vi "TCPtaskhandle.vi"(6 "心跳包":refnum<vi>, 9 "配置信息":refnum<vi>, 10 "状态信息":refnum<vi>, 11 "通信状态":refnum<vi>) -> ()   [LabVIEW 2016, in "数据传输系统-06.lvlib"]
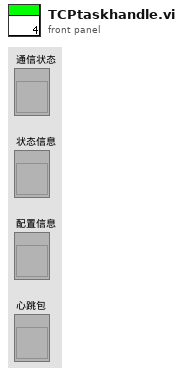
[diagram p1: front panel]
types:
  T1 = cluster{"枚举":enum16{"打开连接", "发送数据", "读取数据", "数据处理", "关闭连接"}, "发送报文":string}
  T2 = cluster{"setini":string, "sysini":string, "hechaini":string, "actualwrite":string, "actualread":string, "datasent":string, "反控命令信息队列":string, "反控与仪器交互":string}
  T3 = cluster{"站点":string, "设备":string, "IP":string, "PORT":string, "MN":string, "PW":string}
  T4 = cluster{"1st Error to Convert ":i32, "步骤 ":enum16{"打开连接", "发送数据", "读取数据", "数据处理", "关闭连接"}, "元素":string, "TCP服务端掉线计数":i32, "TCP掉线时间节点":string}
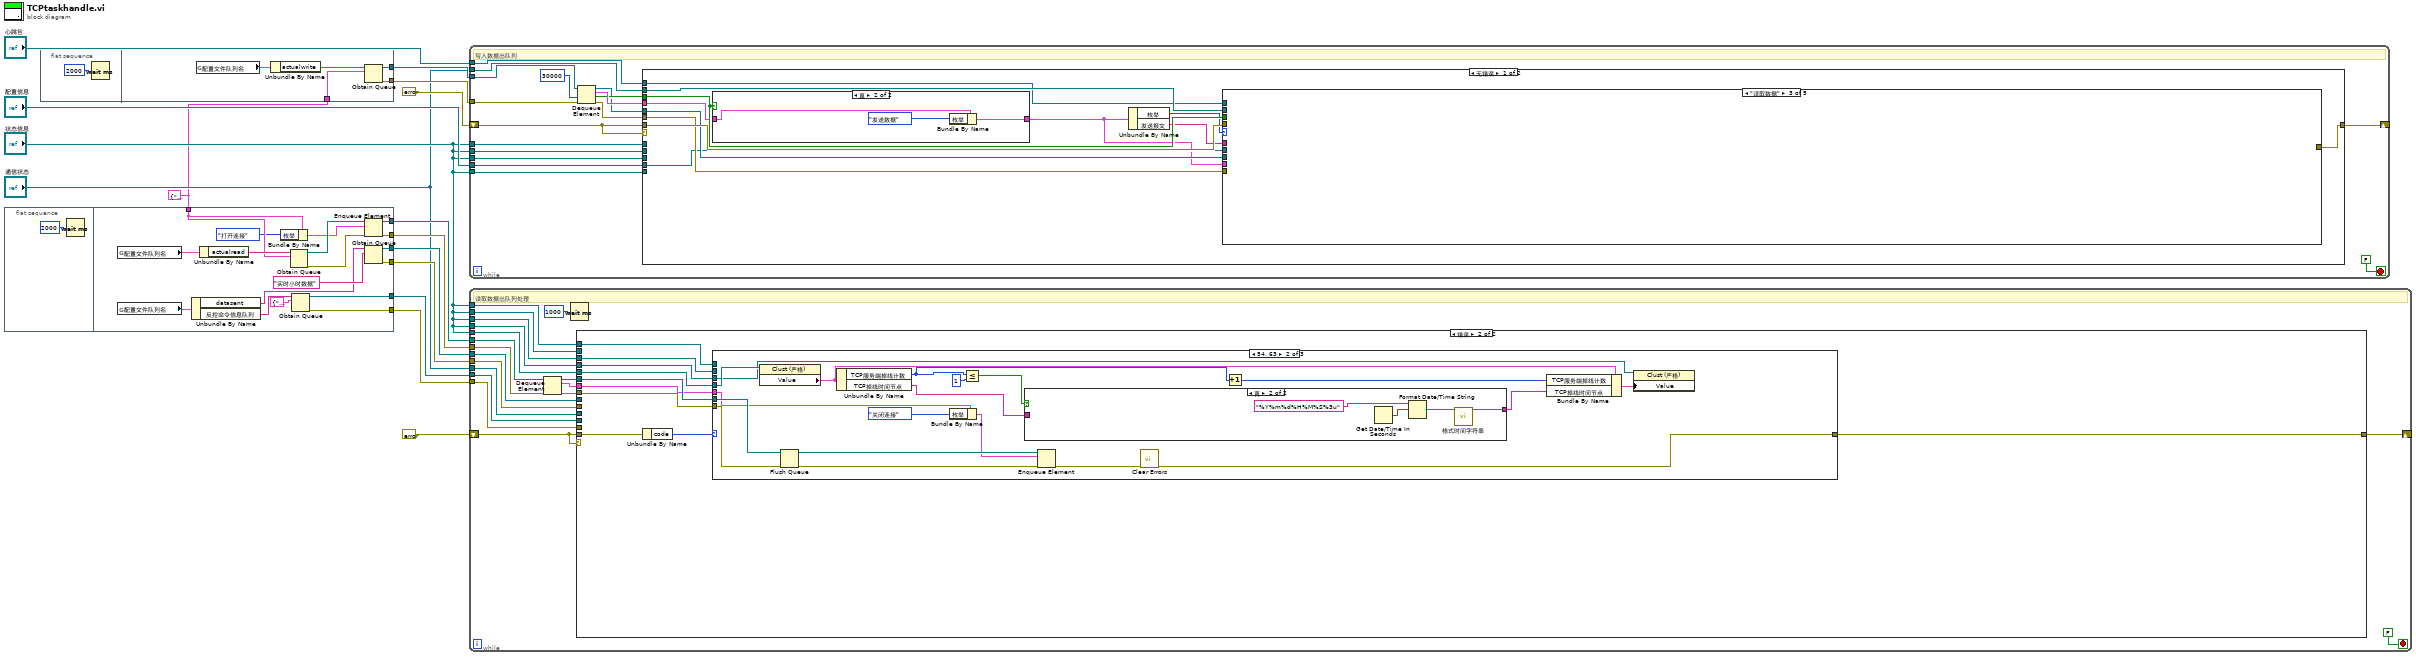
[diagram p0: block diagram]
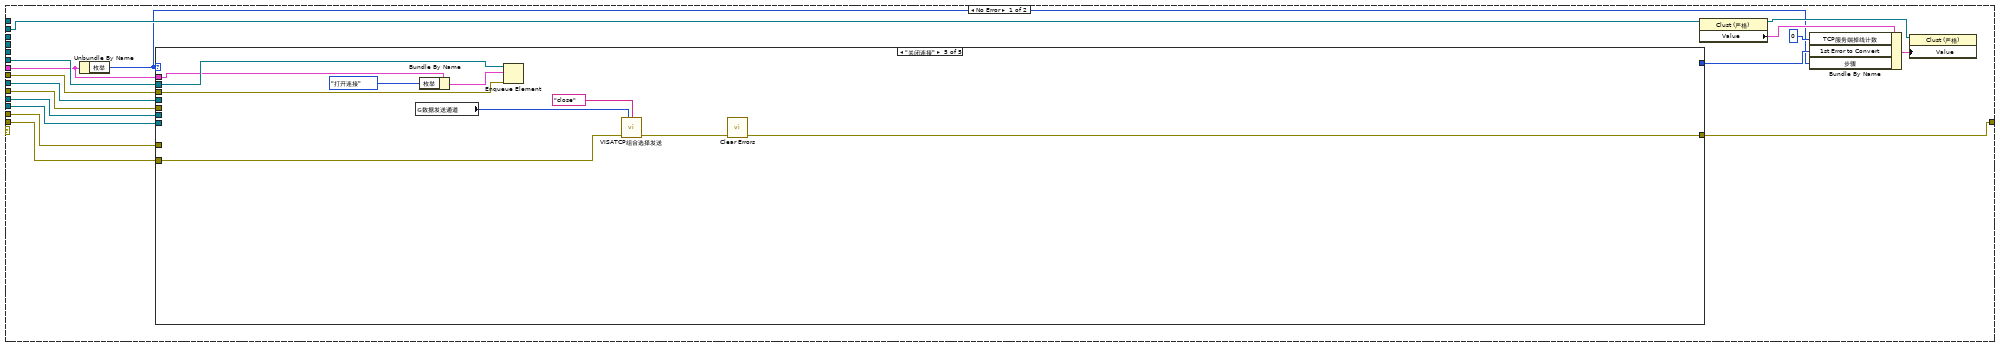
[diagram p2: hidden frame]
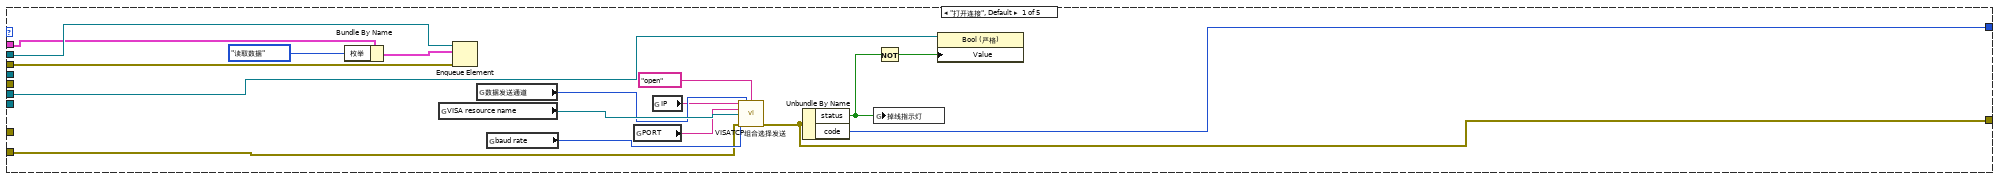
[diagram p3: hidden frame]
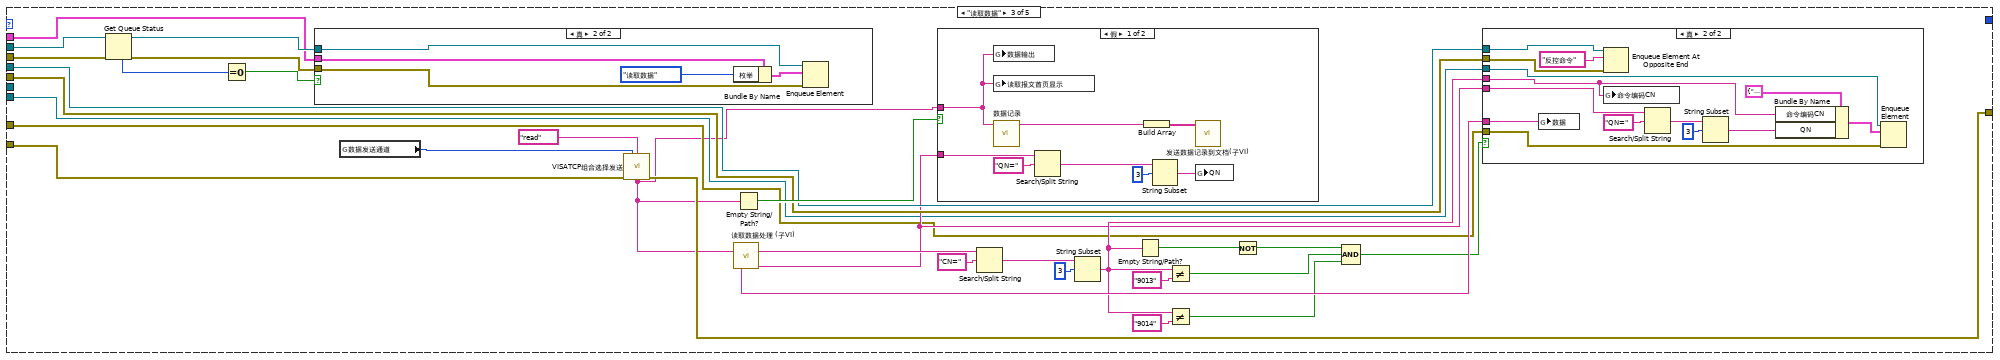
[diagram p5: hidden frame]
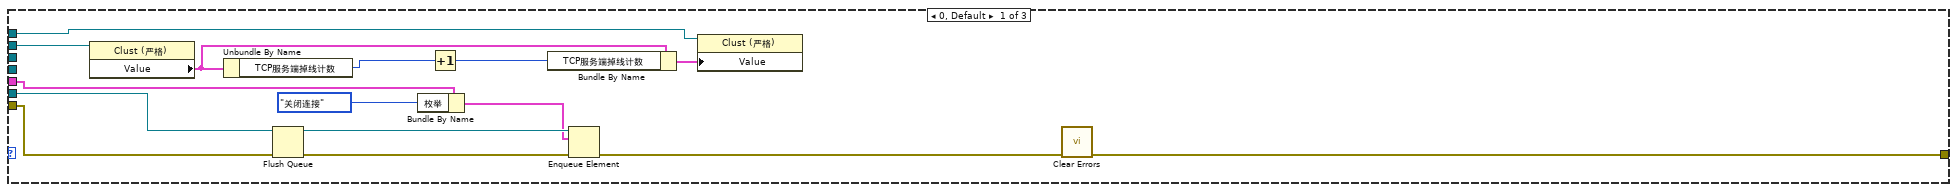
[diagram p10: hidden frame]
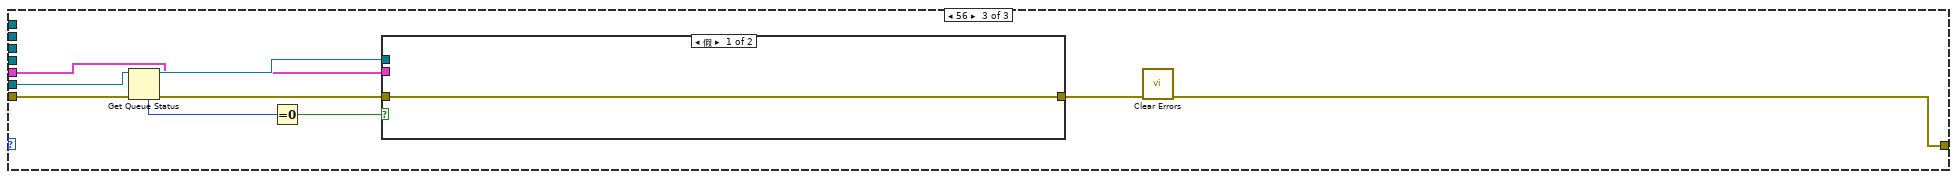
[diagram p12: hidden frame]
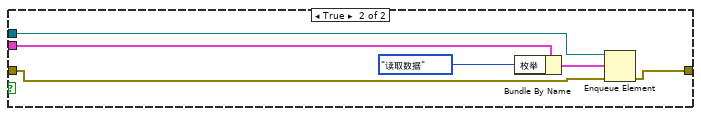
[diagram p13: hidden frame]
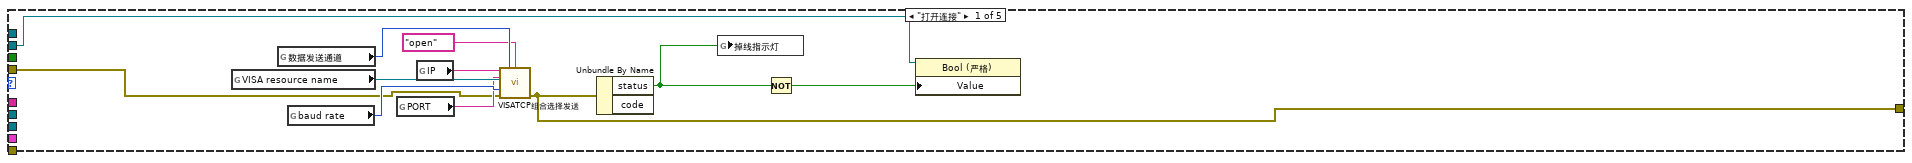
[diagram p14: hidden frame]
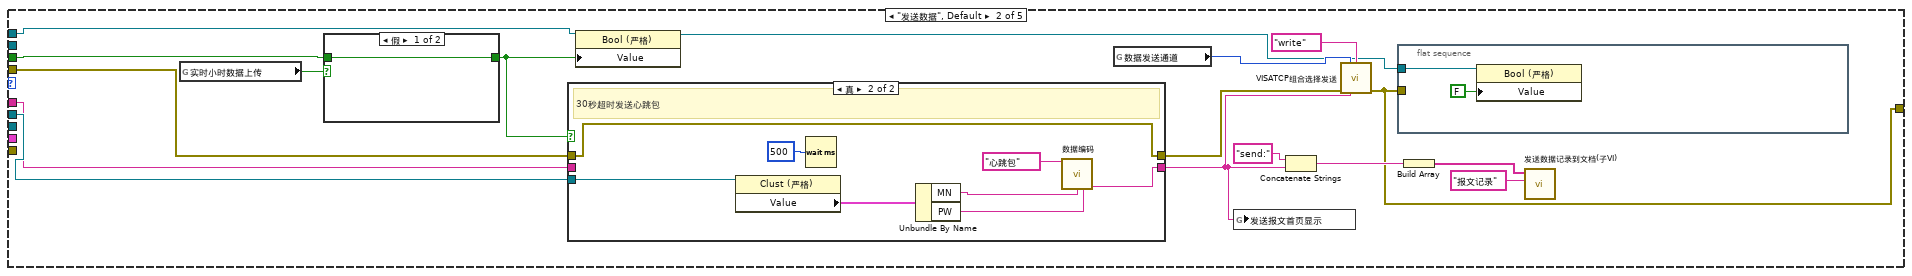
[diagram p15: hidden frame]
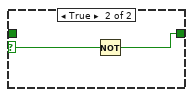
[diagram p17: hidden frame]
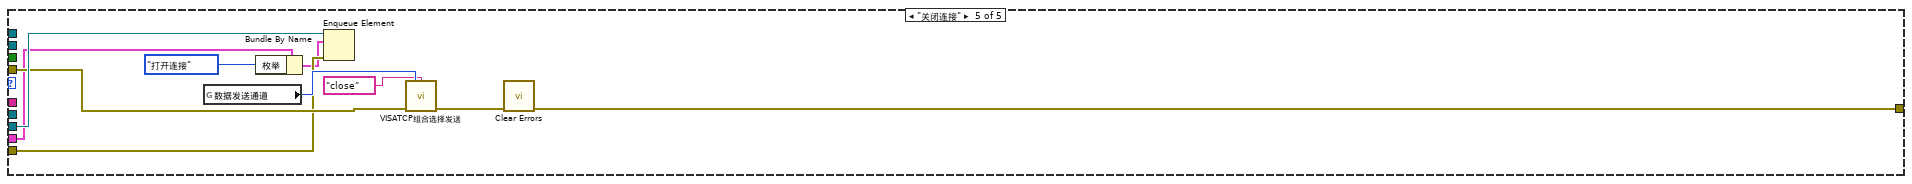
[diagram p19: hidden frame]
diagram:
  w1 = T1 {"枚举"=enum."打开连接", "发送报文"=""} ("data")
  n1 = flat-sequence {
    tunnel: [w33] -> w9
    tunnel: [w32] -> w10
    tunnel: [w30] -> w12
    tunnel: [w29] -> w13
    tunnel: [w27] -> w14
    tunnel: [w26] -> w15
    tunnel: w1 -> [w19]
    frame #0 {
      n2 = Wait (ms)(milliseconds to wait=u32 2000 ("等待时间（毫秒）")) -> ()  [unwired: 1 out]
    }
    frame #1 {
      n3 = global read "断电保存全局.vi" "配置文件队列名"() -> (w24:T2)
      n4 = global read "断电保存全局.vi" "配置文件队列名"() -> (w22:T2)
      n5 = Unbundle By Name(w22) -> ("datasent"=w21:string, "反控命令信息队列"=w20:string)
      n6 = Unbundle By Name(w24) -> ("actualread"=w23:string)
      n7 = Bundle By Name(cluster=w19, "枚举"=enum16{"打开连接", "发送数据", "读取数据", "数据处理", "关闭连接"}."打开连接") -> (w17:T1)
      n8 = Obtain Queue(name (unnamed)=w23, element data type=w19) -> (queue out=w34:refnum<queue>, error out=w31:errorcluster)  [unwired: 3 in, 1 out]
      n9 = Obtain Queue(name (unnamed)=w20, element data type=cluster{"命令编码CN":string, "QN":string} {"命令编码CN"="", "QN"=""}) -> (queue out=w27:refnum<queue>, error out=w26:errorcluster)  [unwired: 3 in, 1 out]
      n10 = Enqueue Element(queue=w34, element=w17, error in (no error)=w31) -> (queue out=w33:refnum<queue>, error out=w32:errorcluster)  [unwired: 1 in, 1 out]
      n11 = Obtain Queue(name (unnamed)=w21, element data type="实时小时数据" ("元素")) -> (queue out=w30:refnum<queue>, error out=w29:errorcluster)  [unwired: 3 in, 1 out]
    }
  }
  n12 = flat-sequence {
    tunnel: [w40] -> w6
    tunnel: [w39] -> w7
    tunnel: w1 -> [w36]
    frame #0 {
      n13 = Wait (ms)(milliseconds to wait=u32 2000 ("等待时间（毫秒）")) -> ()  [unwired: 1 out]
    }
    frame #1 {
      n14 = global read "断电保存全局.vi" "配置文件队列名"() -> (w38:T2)
      n15 = Unbundle By Name(w38) -> ("actualwrite"=w37:string)
      n16 = Obtain Queue(name (unnamed)=w37, element data type=w36) -> (queue out=w40:refnum<queue>, error out=w39:errorcluster)  [unwired: 3 in, 1 out]
    }
  }
  n17 = while {
    tunnel: w6 -> [w56]
    tunnel: w7 -> [w55]
    shift-right: [w51] -> _
    shift-left: errorcluster {"status"=FALSE, "code"=0, "source"=""} ("error out") -> [w50]
    tunnel: "通信状态" -> [w47]
    tunnel: "配置信息" -> [w46]
    tunnel: "心跳包" -> [w45]
    tunnel: "状态信息" -> [w44]
    tunnel: "状态信息" -> [w43]
    tunnel: "状态信息" -> [w42]
    tunnel: "状态信息" -> [w41]
    stop <- FALSE stop-if-true
    # "写入数据出队列"
    n18 = Dequeue Element(queue=w56, timeout in ms (-1)=30000 ("超时毫秒(-1)"), error in (no error)=w55) -> (queue out=w49:refnum<queue>, element=w53:T1, timed out?=w52:bool, error out=w48:errorcluster)
    n19 = case shown="无错误" w50 {
      tunnel: w53 -> [w64 w127]
      tunnel: w52 -> [w65 _]
      tunnel: [w69 w132] -> w51
      tunnel: w50 -> [w68 w136]
      tunnel: w49 -> [w67 w134]
      tunnel: w48 -> [w66 w133]
      tunnel: w47 -> [w63 _]
      tunnel: w46 -> [w62 _]
      tunnel: w45 -> [w61 _]
      tunnel: w44 -> [_ w131]
      tunnel: w43 -> [_ w130]
      tunnel: w42 -> [_ w129]
      tunnel: w41 -> [_ w128]
      frame No Error {
        n20 = case shown="真" w65 {
          tunnel: [w123 w124] -> w58
          tunnel: w64 -> [w123 w126]
          frame False {
          }
          frame True {
            n21 = Bundle By Name(cluster=w126, "枚举"=enum16{"打开连接", "发送数据", "读取数据", "数据处理", "关闭连接"}."发送数据") -> (w124:T1)
          }
        }
        n22 = Unbundle By Name(w58) -> ("枚举"=w60:enum16{"打开连接", "发送数据", "读取数据", "数据处理", "关闭连接"}, "发送报文"=w59:string)
        n23 = case shown="\"读取数据\"" w60 {
          tunnel: w65 -> [_ w87 _ _ _]
          tunnel: [w72 w90 _ _ w117] -> w69
          tunnel: w68 -> [w74 w95 _ _ w118]
          tunnel: w67 -> [_ _ _ _ w119]
          tunnel: w66 -> [_ _ _ _ w116]
          tunnel: w63 -> [w70 _ _ _ _]
          tunnel: w62 -> [_ w86 _ _ _]
          tunnel: w61 -> [_ w84 _ _ _]
          tunnel: w59 -> [_ w82 _ _ _]
          tunnel: w58 -> [_ _ _ _ w114]
          frame "打开连接" {
            n24 = global read "断电保存全局.vi" "VISA resource name"() -> (w80:refnum<visa-resource-name>)
            n25 = global read "断电保存全局.vi" "数据发送通道"() -> (w77:enum16{"TCP", "VISA"})
            n26 = global read "断电保存全局.vi" "baud rate"() -> (w79:u32)
            n27 = global read "断电保存全局.vi" "PORT"() -> (w78:string)
            n28 = global read "断电保存全局.vi" "IP"() -> (w76:string)
            n29 = call "VISATCP组合选择发送.vi"("IP"=w76, "数据发送通道"=w77, "命令"="open", "PORT"=w78, "VISA resource name"=w80, "baud rate"=w79, "error in (no error)"=w74) -> ("错误输出"=w72:errorcluster)  [unwired: 5 in, 3 out]
            n30 = Unbundle By Name(w72) -> ("status"=w71:bool)  [unwired: 1 out]
            n31 = global write "全局 数据发送重叠.vi" "掉线指示灯"(w71) -> ()
            n32 = Not(x=w71) -> (.not. x?=w73:bool)
            n33 = property class="Bool (严格)"(reference=w70, "Value"=w73) -> ()  [unwired: 1 in, 2 out]
          }
          frame "发送数据", Default {
            n34 = global read "全局1.vi" "实时小时数据上传"() -> (w88:bool)
            n35 = case shown="假" w88 {
              selector: w88 -> [_ w112]
              tunnel: w87 -> [w110 _]
              tunnel: [w110 w111] -> w85
              frame False {
              }
              frame True {
                n36 = Not(x=w112) -> (.not. x?=w111:bool)
              }
            }
            n37 = case shown="真" w85 {
              tunnel: [w100 w104] -> w81
              tunnel: w95 -> [w101 w105]
              tunnel: [w101 w105] -> w94
              tunnel: w86 -> [_ w102]
              tunnel: w82 -> [w100 _]
              frame False {
                # "事件触发发送数据"
              }
              frame True {
                # "30秒超时发送心跳包"
                n38 = property class="Clust (严格)"(reference=w102) -> ("Value"=w108:T3)  [unwired: 1 in, 2 out]
                n39 = Wait (ms)(milliseconds to wait=u32 500 ("等待时间（毫秒）")) -> ()  [unwired: 1 out]
                n40 = Unbundle By Name(w108) -> ("MN"=w107:string, "PW"=w106:string)
                n41 = call "数据编码.vi"("table输入"="心跳包", "MN"=w107, "PW"=w106) -> ("通讯包字符串"=w104:string)  [unwired: 11 in, 1 out]
              }
            }
            n42 = property class="Bool (严格)"(reference=w84, "Value"=w85) -> (reference out=w83:refnum<vi>)  [unwired: 1 in, 1 out]
            n43 = global read "断电保存全局.vi" "数据发送通道"() -> (w96:enum16{"TCP", "VISA"})
            n44 = global write "全局1.vi" "发送报文首页显示"(w81) -> ()
            n45 = Concatenate Strings("send:" ("字符串"), w81) -> (w91:string)
            n46 = call "VISATCP组合选择发送.vi"("数据发送通道"=w96, "命令"="write", "error in (no error)"=w94, "写入缓冲区"=w81) -> ("错误输出"=w90:errorcluster)  [unwired: 8 in, 3 out]
            n47 = flat-sequence {
              tunnel: w90 -> [_]
              tunnel: w83 -> [w98]
              frame #0 {
                n48 = property class="Bool (严格)"(reference=w98, "Value"=FALSE ("心跳包")) -> ()  [unwired: 1 in, 2 out]
              }
            }
            n49 = Build Array(w91) -> (w93:string[])
            n50 = call "发送数据记录到文档(子VI).vi"("字符串"="报文记录", "数组"=w93) -> ()  [unwired: 8 in, 1 out]
          }
          frame "读取数据" {
          }
          frame "数据处理" {
          }
          frame "关闭连接" {
            n51 = global read "断电保存全局.vi" "数据发送通道"() -> (w121:enum16{"TCP", "VISA"})
            n52 = Bundle By Name(cluster=w114, "枚举"=enum16{"打开连接", "发送数据", "读取数据", "数据处理", "关闭连接"}."打开连接") -> (w113:T1)
            n53 = Enqueue Element(queue=w119, element=w113, error in (no error)=w116) -> ()  [unwired: 1 in, 3 out]
            n54 = call "VISATCP组合选择发送.vi"("数据发送通道"=w121, "命令"="close", "error in (no error)"=w118) -> ("错误输出"=w122:errorcluster)  [unwired: 9 in, 3 out]
            n55 = call <vilib>:"Clear Errors.vi"("error in (no error)"=w122) -> ("error out"=w117:errorcluster)  [unwired: 5 in, 1 out]
          }
        }
      }
      frame Error {
        n56 = Unbundle By Name(w136) -> ("code"=w135:i32)
        n57 = case shown="0, 默认" w135 {
          tunnel: w134 -> [w148 w168 w179]
          tunnel: w133 -> [w147 w167 w178]
          tunnel: [w146 w165 w177] -> w132
          tunnel: w131 -> [w141 _ _]
          tunnel: w130 -> [w140 _ _]
          tunnel: w129 -> [_ w156 _]
          tunnel: w128 -> [_ w155 _]
          tunnel: w127 -> [w138 w154 _]
          frame 0, Default {
            n58 = property class="Clust (严格)"(reference=w141) -> ("Value"=w145:T4)  [unwired: 1 in, 2 out]
            n59 = Unbundle By Name(w145) -> ("TCP服务端掉线计数"=w143:i32)
            n60 = Flush Queue(queue=w148, error in (no error)=w147) -> (queue out=w149:refnum<queue>, error out=w150:errorcluster)  [unwired: 1 out]
            n61 = Bundle By Name(cluster=w138, "枚举"=enum16{"打开连接", "发送数据", "读取数据", "数据处理", "关闭连接"}."关闭连接") -> (w137:T1)
            n62 = Increment(x=w143) -> (x+1=w144:i32)
            n63 = Bundle By Name(cluster=w145, "TCP服务端掉线计数"=w144) -> (w142:T4)
            n64 = Enqueue Element(queue=w149, element=w137, error in (no error)=w150) -> (error out=w151:errorcluster)  [unwired: 1 in, 2 out]
            n65 = property class="Clust (严格)"(reference=w140, "Value"=w142) -> ()  [unwired: 1 in, 2 out]
            n66 = call <vilib>:"Clear Errors.vi"("error in (no error)"=w151) -> ("error out"=w146:errorcluster)  [unwired: 5 in, 1 out]
          }
          frame 54, 63 {
            n67 = property class="Clust (严格)"(reference=w156) -> ("Value"=w160:T4)  [unwired: 1 in, 2 out]
            n68 = Flush Queue(queue=w168, error in (no error)=w167) -> (queue out=w169:refnum<queue>, error out=w170:errorcluster)  [unwired: 1 out]
            n69 = Unbundle By Name(w160) -> ("TCP服务端掉线计数"=w164:i32, "TCP掉线时间节点"=w157:string)
            n70 = Bundle By Name(cluster=w154, "枚举"=enum16{"打开连接", "发送数据", "读取数据", "数据处理", "关闭连接"}."关闭连接") -> (w152:T1)
            n71 = Less Or Equal?(x=w164, y=1) -> (x <= y?=w162:bool)
            n72 = case shown="真" w162 {
              tunnel: [w171 w172] -> w161
              tunnel: w157 -> [w171 _]
              frame False {
              }
              frame True {
                n73 = Get Date/Time In Seconds() -> (seconds since 1Jan1904=w173:timestamp)
                n74 = Format Date/Time String(time format string (%c)="%Y%m%d%H%M%S%3u" ("时间格式字符串(%c)"), seconds (now)=w173) -> (date/time string=w175:string)  [unwired: 1 in]
                n75 = call "格式时间字符串.vi"("字符串"=w175) -> ("连接的字符串"=w172:string)  [unwired: 10 in]
              }
            }
            n76 = Enqueue Element(queue=w169, element=w152, error in (no error)=w170) -> (error out=w166:errorcluster)  [unwired: 1 in, 2 out]
            n77 = call <vilib>:"Clear Errors.vi"("error in (no error)"=w166) -> ("error out"=w165:errorcluster)  [unwired: 5 in, 1 out]
            n78 = Increment(x=w164) -> (x+1=w159:i32)
            n79 = Bundle By Name(cluster=w160, "TCP服务端掉线计数"=w159, "TCP掉线时间节点"=w161) -> (w158:T4)
            n80 = property class="Clust (严格)"(reference=w155, "Value"=w158) -> ()  [unwired: 1 in, 2 out]
          }
          frame 56 {
            n81 = Flush Queue(queue=w179, error in (no error)=w178) -> (error out=w176:errorcluster)  [unwired: 2 out]
            n82 = call <vilib>:"Clear Errors.vi"("error in (no error)"=w176) -> ("error out"=w177:errorcluster)  [unwired: 5 in, 1 out]
          }
        }
      }
    }
  }
  n83 = while {
    tunnel: w9 -> [w198]
    tunnel: w10 -> [w197]
    shift-right: [w194] -> _
    shift-left: errorcluster {"status"=FALSE, "code"=0, "source"=""} ("error out") -> [w193]
    tunnel: w12 -> [w189]
    tunnel: w13 -> [w188]
    tunnel: w14 -> [w187]
    tunnel: w15 -> [w186]
    tunnel: "状态信息" -> [w185]
    tunnel: "状态信息" -> [w184]
    tunnel: "状态信息" -> [w183]
    tunnel: "状态信息" -> [w182]
    tunnel: "状态信息" -> [w181]
    tunnel: "通信状态" -> [w180]
    stop <- FALSE stop-if-true
    # "读取数据出队列处理"
    n84 = Dequeue Element(queue=w198, error in (no error)=w197) -> (queue out=w192:refnum<queue>, element=w195:T1, error out=w191:errorcluster)  [unwired: 1 in, 1 out]
    n85 = Wait (ms)(milliseconds to wait=u32 1000 ("等待时间（毫秒）")) -> ()  [unwired: 1 out]
    n86 = case shown="错误" w193 {
      tunnel: w195 -> [w199 w301]
      tunnel: [w215 w306] -> w194
      tunnel: w193 -> [w214 w310]
      tunnel: w192 -> [w213 w308]
      tunnel: w191 -> [w212 w307]
      tunnel: w189 -> [w208 _]
      tunnel: w188 -> [w207 _]
      tunnel: w187 -> [w206 _]
      tunnel: w186 -> [w205 _]
      tunnel: w185 -> [w204 _]
      tunnel: w184 -> [_ w305]
      tunnel: w183 -> [_ w304]
      tunnel: w182 -> [_ w303]
      tunnel: w181 -> [_ w302]
      tunnel: w180 -> [w201 _]
      frame No Error {
        n87 = Unbundle By Name(w199) -> ("枚举"=w200:enum16{"打开连接", "发送数据", "读取数据", "数据处理", "关闭连接"})
        n88 = case shown="\"关闭连接\"" w200 {
          tunnel: [w226 _ w260 _ w296] -> w215
          tunnel: w214 -> [w225 _ w263 _ w297]
          tunnel: w213 -> [w224 _ w255 _ w295]
          tunnel: w212 -> [w223 _ w254 _ w294]
          tunnel: [w222 _ _ _ _] -> w210
          tunnel: w208 -> [_ _ w248 _ _]
          tunnel: w207 -> [_ _ w247 _ _]
          tunnel: w206 -> [_ _ w236 _ _]
          tunnel: w205 -> [_ _ w235 _ _]
          tunnel: w201 -> [w220 _ _ _ _]
          tunnel: w199 -> [w217 _ w233 _ w291]
          frame "打开连接", Default {
            n89 = Bundle By Name(cluster=w217, "枚举"=enum16{"打开连接", "发送数据", "读取数据", "数据处理", "关闭连接"}."读取数据") -> (w216:T1)
            n90 = global read "断电保存全局.vi" "VISA resource name"() -> (w232:refnum<visa-resource-name>)
            n91 = Enqueue Element(queue=w224, element=w216, error in (no error)=w223) -> ()  [unwired: 1 in, 3 out]
            n92 = global read "断电保存全局.vi" "数据发送通道"() -> (w229:enum16{"TCP", "VISA"})
            n93 = global read "断电保存全局.vi" "baud rate"() -> (w231:u32)
            n94 = global read "断电保存全局.vi" "PORT"() -> (w230:string)
            n95 = global read "断电保存全局.vi" "IP"() -> (w228:string)
            n96 = call "VISATCP组合选择发送.vi"("IP"=w228, "数据发送通道"=w229, "命令"="open", "PORT"=w230, "VISA resource name"=w232, "baud rate"=w231, "error in (no error)"=w225) -> ("错误输出"=w226:errorcluster)  [unwired: 5 in, 3 out]
            n97 = Unbundle By Name(w226) -> ("status"=w221:bool, "code"=w222:i32)
            n98 = global write "全局 数据发送重叠.vi" "掉线指示灯"(w221) -> ()
            n99 = Not(x=w221) -> (.not. x?=w219:bool)
            n100 = property class="Bool (严格)"(reference=w220, "Value"=w219) -> ()  [unwired: 1 in, 2 out]
          }
          frame "发送数据" {
          }
          frame "读取数据" {
            n101 = Get Queue Status(queue=w255, error in (no error)=w254) -> (queue out=w251:refnum<queue>, error out=w250:errorcluster, # elements in queue=w253:i32)  [unwired: 1 in, 5 out]
            n102 = Equal To 0?(x=w253) -> (x = 0?=w252:bool)
            n103 = case shown="真" w252 {
              tunnel: w251 -> [_ w290]
              tunnel: w250 -> [_ w289]
              tunnel: w233 -> [_ w288]
              frame False {
              }
              frame True {
                n104 = Bundle By Name(cluster=w288, "枚举"=enum16{"打开连接", "发送数据", "读取数据", "数据处理", "关闭连接"}."读取数据") -> (w286:T1)
                n105 = Enqueue Element(queue=w290, element=w286, error in (no error)=w289) -> ()  [unwired: 1 in, 3 out]
              }
            }
            n106 = global read "断电保存全局.vi" "数据发送通道"() -> (w262:enum16{"TCP", "VISA"})
            n107 = call "VISATCP组合选择发送.vi"("数据发送通道"=w262, "命令"="read", "error in (no error)"=w263) -> ("读取缓冲区"=w234:string, "错误输出"=w260:errorcluster)  [unwired: 9 in, 2 out]
            n108 = call "读取数据处理 (子VI).vi"("data out"=w234) -> ("命令编码CN"=w256:string, "数据"=w245:string, "时间QN"=w237:string)  [unwired: 8 in, 4 out]
            n109 = Empty String/Path?(string/path=w234) -> (empty?=w249:bool)
            n110 = case shown="假" w249 {
              tunnel: w234 -> [w283 _]
              tunnel: w237 -> [w280 _]
              frame False {
                n111 = global write "全局1.vi" "数据输出"(w283) -> ()
                n112 = global write "全局1.vi" "读取报文首页显示"(w283) -> ()
                n113 = call "数据记录.vi"("写入字段"=w283) -> ("连接的字符串"=w284:string)  [unwired: 10 in]
                n114 = Search/Split String(string=w280, search string/char (-)="QN=" ("搜索字符串/字符(-)")) -> (match + rest of string=w279:string)  [unwired: 1 in, 2 out]
                n115 = Build Array(w284) -> (w285:string[])
                n116 = String Subset(string=w279, offset (0)=3 ("偏移量(0)")) -> (substring=w278:string)  [unwired: 1 in]
                n117 = call "发送数据记录到文档(子VI).vi"("数组"=w285) -> ()  [unwired: 9 in, 1 out]
                n118 = global write "全局1.vi" "QN"(w278) -> ()
              }
              frame True {
              }
            }
            n119 = Search/Split String(string=w256, search string/char (-)="CN=" ("搜索字符串/字符(-)")) -> (match + rest of string=w257:string)  [unwired: 1 in, 2 out]
            n120 = String Subset(string=w257, offset (0)=3 ("偏移量(0)")) -> (substring=w243:string)  [unwired: 1 in]
            n121 = Empty String/Path?(string/path=w243) -> (empty?=w246:bool)
            n122 = Not Equal?(x=w243, y="9013") -> (x != y?=w240:bool)
            n123 = Not Equal?(x=w243, y="9014") -> (x != y?=w239:bool)
            n124 = Not(x=w246) -> (.not. x?=w238:bool)
            n125 = Compound Arithmetic op=AND ("复合运算")(w238, w240, w239) -> (w244:bool)
            n126 = case shown="真" w244 {
              tunnel: w248 -> [_ w277]
              tunnel: w247 -> [_ w276]
              tunnel: w245 -> [_ w275]
              tunnel: w243 -> [_ w266]
              tunnel: w237 -> [_ w271]
              tunnel: w236 -> [_ w270]
              tunnel: w235 -> [_ w269]
              frame False {
              }
              frame True {
                n127 = global write "全局1.vi" "数据"(w275) -> ()
                n128 = Enqueue Element At Opposite End(queue=w277, element="反控命令" ("元素"), error in (no error)=w276) -> ()  [unwired: 1 in, 3 out]
                n129 = global write "全局1.vi" "命令编码CN"(w266) -> ()
                n130 = Search/Split String(string=w271, search string/char (-)="QN=" ("搜索字符串/字符(-)")) -> (match + rest of string=w274:string)  [unwired: 1 in, 2 out]
                n131 = String Subset(string=w274, offset (0)=3 ("偏移量(0)")) -> (substring=w265:string)  [unwired: 1 in]
                n132 = Bundle By Name(cluster=cluster{"命令编码CN":string, "QN":string} {"命令编码CN"="", "QN"=""}, "命令编码CN"=w266, "QN"=w265) -> (w267:cluster{"命令编码CN":string, "QN":string})
                n133 = Enqueue Element(queue=w270, element=w267, error in (no error)=w269) -> ()  [unwired: 1 in, 3 out]
              }
            }
          }
          frame "数据处理" {
          }
          frame "关闭连接" {
            n134 = global read "断电保存全局.vi" "数据发送通道"() -> (w299:enum16{"TCP", "VISA"})
            n135 = Bundle By Name(cluster=w291, "枚举"=enum16{"打开连接", "发送数据", "读取数据", "数据处理", "关闭连接"}."打开连接") -> (w292:T1)
            n136 = Enqueue Element(queue=w295, element=w292, error in (no error)=w294) -> ()  [unwired: 1 in, 3 out]
            n137 = call "VISATCP组合选择发送.vi"("数据发送通道"=w299, "命令"="close", "error in (no error)"=w297) -> ("错误输出"=w298:errorcluster)  [unwired: 9 in, 3 out]
            n138 = call <vilib>:"Clear Errors.vi"("error in (no error)"=w298) -> ("error out"=w296:errorcluster)  [unwired: 5 in, 1 out]
          }
        }
        n139 = property class="Clust (严格)"(reference=w204) -> (reference out=w203:refnum<vi>, "Value"=w211:T4)  [unwired: 1 in, 1 out]
        n140 = Bundle By Name(cluster=w211, "TCP服务端掉线计数"=0, "1st Error to Convert"=w210, "步骤"=w200) -> (w202:T4)
        n141 = property class="Clust (严格)"(reference=w203, "Value"=w202) -> ()  [unwired: 1 in, 2 out]
      }
      frame Error {
        n142 = Unbundle By Name(w310) -> ("code"=w309:i32)
        n143 = case shown="54, 63" w309 {
          tunnel: w308 -> [w322 w342 w352]
          tunnel: w307 -> [w321 w341 w351]
          tunnel: [w320 w339 w358] -> w306
          tunnel: w305 -> [w315 _ _]
          tunnel: w304 -> [w314 _ _]
          tunnel: w303 -> [_ w330 _]
          tunnel: w302 -> [_ w329 _]
          tunnel: w301 -> [w313 w328 w350]
          frame 0, Default {
            n144 = property class="Clust (严格)"(reference=w315) -> ("Value"=w319:T4)  [unwired: 1 in, 2 out]
            n145 = Unbundle By Name(w319) -> ("TCP服务端掉线计数"=w317:i32)
            n146 = Flush Queue(queue=w322, error in (no error)=w321) -> (queue out=w323:refnum<queue>, error out=w324:errorcluster)  [unwired: 1 out]
            n147 = Bundle By Name(cluster=w313, "枚举"=enum16{"打开连接", "发送数据", "读取数据", "数据处理", "关闭连接"}."关闭连接") -> (w311:T1)
            n148 = Increment(x=w317) -> (x+1=w318:i32)
            n149 = Bundle By Name(cluster=w319, "TCP服务端掉线计数"=w318) -> (w316:T4)
            n150 = Enqueue Element(queue=w323, element=w311, error in (no error)=w324) -> (error out=w325:errorcluster)  [unwired: 1 in, 2 out]
            n151 = property class="Clust (严格)"(reference=w314, "Value"=w316) -> ()  [unwired: 1 in, 2 out]
            n152 = call <vilib>:"Clear Errors.vi"("error in (no error)"=w325) -> ("error out"=w320:errorcluster)  [unwired: 5 in, 1 out]
          }
          frame 54, 63 {
            n153 = property class="Clust (严格)"(reference=w330) -> ("Value"=w334:T4)  [unwired: 1 in, 2 out]
            n154 = Flush Queue(queue=w342, error in (no error)=w341) -> (queue out=w343:refnum<queue>, error out=w344:errorcluster)  [unwired: 1 out]
            n155 = Unbundle By Name(w334) -> ("TCP服务端掉线计数"=w338:i32, "TCP掉线时间节点"=w331:string)
            n156 = Bundle By Name(cluster=w328, "枚举"=enum16{"打开连接", "发送数据", "读取数据", "数据处理", "关闭连接"}."关闭连接") -> (w326:T1)
            n157 = Less Or Equal?(x=w338, y=1) -> (x <= y?=w336:bool)
            n158 = case shown="真" w336 {
              tunnel: [w345 w346] -> w335
              tunnel: w331 -> [w345 _]
              frame False {
              }
              frame True {
                n159 = Get Date/Time In Seconds() -> (seconds since 1Jan1904=w347:timestamp)
                n160 = Format Date/Time String(time format string (%c)="%Y%m%d%H%M%S%3u" ("时间格式字符串(%c)"), seconds (now)=w347) -> (date/time string=w349:string)  [unwired: 1 in]
                n161 = call "格式时间字符串.vi"("字符串"=w349) -> ("连接的字符串"=w346:string)  [unwired: 10 in]
              }
            }
            n162 = Enqueue Element(queue=w343, element=w326, error in (no error)=w344) -> (error out=w340:errorcluster)  [unwired: 1 in, 2 out]
            n163 = call <vilib>:"Clear Errors.vi"("error in (no error)"=w340) -> ("error out"=w339:errorcluster)  [unwired: 5 in, 1 out]
            n164 = Increment(x=w338) -> (x+1=w333:i32)
            n165 = Bundle By Name(cluster=w334, "TCP服务端掉线计数"=w333, "TCP掉线时间节点"=w335) -> (w332:T4)
            n166 = property class="Clust (严格)"(reference=w329, "Value"=w332) -> ()  [unwired: 1 in, 2 out]
          }
          frame 56 {
            n167 = Get Queue Status(queue=w352, error in (no error)=w351) -> (queue out=w354:refnum<queue>, error out=w353:errorcluster, # elements in queue=w356:i32)  [unwired: 1 in, 5 out]
            n168 = Equal To 0?(x=w356) -> (x = 0?=w355:bool)
            n169 = case shown="假" w355 {
              tunnel: [w359 w365] -> w357
              tunnel: w354 -> [_ w364]
              tunnel: w353 -> [w359 w363]
              tunnel: w350 -> [_ w361]
              frame False {
              }
              frame True {
                n170 = Bundle By Name(cluster=w361, "枚举"=enum16{"打开连接", "发送数据", "读取数据", "数据处理", "关闭连接"}."读取数据") -> (w360:T1)
                n171 = Enqueue Element(queue=w364, element=w360, error in (no error)=w363) -> (error out=w365:errorcluster)  [unwired: 1 in, 2 out]
              }
            }
            n172 = call <vilib>:"Clear Errors.vi"("error in (no error)"=w357) -> ("error out"=w358:errorcluster)  [unwired: 5 in, 1 out]
          }
        }
      }
    }
  }
